vi "Set Version.vi"(8 "error in (no error)":errorcluster, 10 "version":T1, 11 "system in":refnum<class "Systems.lvclass">) -> (0 "error out":errorcluster, 3 "system out":refnum<class "Systems.lvclass">)   [LabVIEW 2013, in "PL Framework Configuration Tool.lvlib" / "Systems.lvclass"]
uses:
  Systems.lvclass
  Systems.lvclass/Systems.ctl
  Framework Configuration Classes/system configuration/PL_System Configuration.lvclass/PL_System Configuration.ctl
  Framework Configuration Classes/system configuration/PL_System Configuration.lvclass
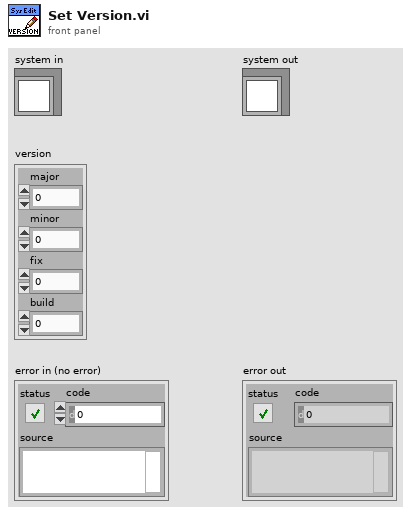
[diagram p1: front panel]
types:
  T1 = cluster{"major":u16, "minor":u16, "fix":u16, "build":u16}
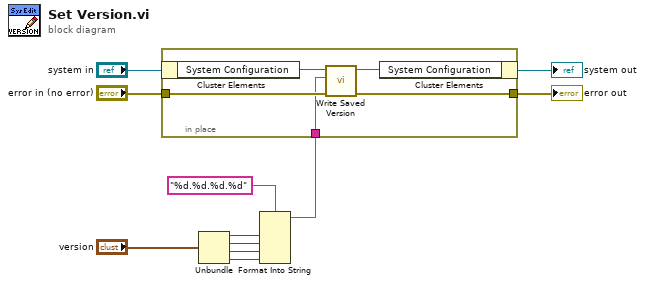
[diagram p0: block diagram]
diagram:
  n1 = Unbundle("version") -> ("major"=w6:u16, "minor"=w5:u16, "fix"=w4:u16, "build"=w3:u16)
  n2 = Format Into String(format string="%d.%d.%d.%d", w6, w5, w4, w3) -> (resulting string=w2:string)  [unwired: 2 in, 1 out]
  n3 = in-place {
    in-place-border: "error in (no error)" -> [w15]
    in-place-border: [w14] -> w1
    in-place-border: w2 -> [w12]
    n4 = in-place-cluster #1("system in") -> ("System Configuration"=w16:refnum<class "PL_System Configuration.lvclass">)
    n5 = call "Write Saved Version.vi"("error in"=w15, "Saved Version"=w12, "PL_System Configuration in"=w16) -> ("error out"=w14:errorcluster, "PL_System Configuration out"=w13:refnum<class "PL_System Configuration.lvclass">)  [unwired: 7 in]
    n6 = in-place-cluster #1("System Configuration"=w13) -> (→"system out":refnum<class "Systems.lvclass">)
  }
  "error out" <- w1
